vi "Accelerometer Angle.vi"() -> ()   [LabVIEW 2025]
doc: "Accelerometer Example\n\nThis example shows how to use a two axis analog accelerometer to measure angle. The angle of rotation is calculated by taking the inverse tangent of the x-axis value (opposite) over the y-axis value (adjacent). This example does not account for the possible inconsistencies within the accelerometer. The calculation is performed assuming the x-axis and y-axis values form a perfect unit circle.\n\nThis example expects a USB cable connected from your development PC to the Type B USB Jack (next to the power input) on the roboRIO."
uses:
  <vilib>/Rock Robotics/WPI/Accelerometer/WPI_AccelerometerScaling.ctl
  <vilib>/Rock Robotics/WPI/Accelerometer/WPI_AccelerometerAnalogChannels.ctl
  <vilib>/Rock Robotics/SystemInterfaces/AI/FPGA_AIChannel.ctl
  <vilib>/Rock Robotics/WPI/Accelerometer/WPI_AccelerometerAnalogOpen.vi
panel:
  in  "Analog Channels":T1={"X-Axis"=enum."AI 0", "Y-Axis"=enum."AI 1", "Z-Axis"=enum."Invalid"}
  in  "Scaling":T3={"Gain (VoltsPerG)"=1.0, "Center Voltage"=2.5}
  out "Degrees of Rotation":dbl(knob) scale=180.0..-180.0
  in  "stop":bool
  out "Accelerometer Chart":cluster{"Acceleration":dbl, "Acceleration":dbl}(graph)
  # "Set these inputs before running."
  # "If the X axis and Y axis accelerometers are at 90 degrees to each other.  And if they have matching sensitivities.  Then geometry can show that tan(a) = x/y."
  # "This dial illustrates the rotation angle (in degrees) of the x-axis of the accelerometer."
  # "X"
  # "Y"
  # "5"
  # "5"
  # "accelerometer pins"
  # "G"
  # "G"
  # "Y axis"
  # "X axis"
  # "y"
  # "x"
  # "a"
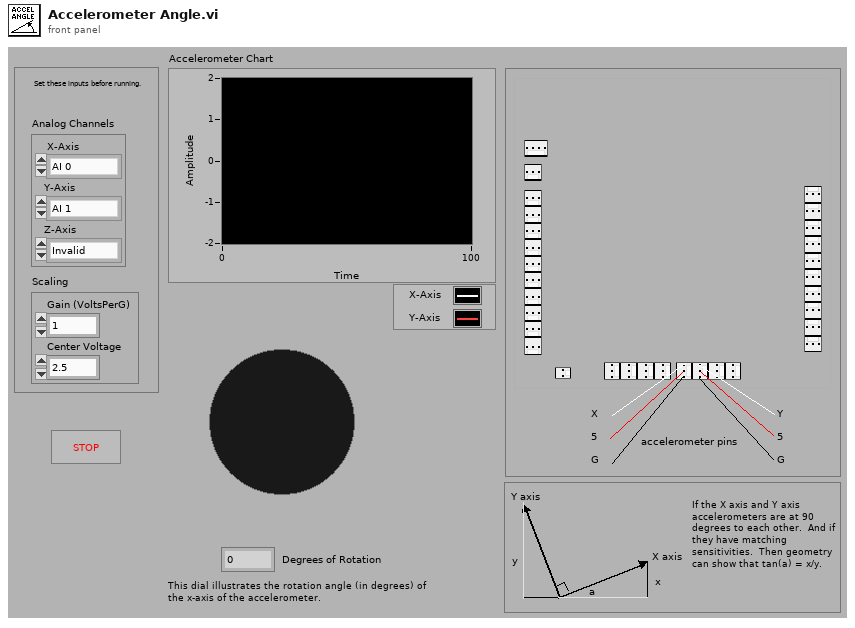
[diagram p1: front panel]
types:
  T1 = typedef "WPI_AccelerometerAnalogChannels.ctl" = cluster{"X-Axis":T2, "Y-Axis":T2, "Z-Axis":T2}
  T2 = typedef "FPGA_AIChannel.ctl" = enum8{"AI 0", "AI 1", "AI 2", "AI 3", "AI MXP 0", "AI MXP 1", "AI MXP 2", "AI MXP 3", "Invalid"}
  T3 = typedef "WPI_AccelerometerScaling.ctl" = cluster{"Gain (VoltsPerG)":dbl, "Center Voltage":dbl}
  T4 = typedef "WPI_AccelerometerDevRef.ctl" = cluster{"DevStatus":errorcluster, "Scaling":T3, "Analog Channels":T1, "I2C Bus":T5, "SPI Bus":T6, "Accel Range":T7, "ADXL Axes":T8, "Handle":i32, "Device Address":u8, "Accel Type":enum16{"Analog", "ADXL345 I2C", "ADXL345 SPI", "Internal", "ADXL362 SPI"}}
  T5 = typedef "i2c_bus.ctl" = enum16{"I2C On-Board", "I2C MXP", "Invalid"}
  T6 = typedef "spi_bus.ctl" = enum16{"SPI On-Board, CS0", "SPI On-Board, CS1", "SPI On-Board, CS2", "SPI On-Board, CS3", "SPI MXP", "Invalid"}
  T7 = typedef "ADXL345 Range.ctl" = u8
  T8 = typedef "WPI_AccelerometerADXL345 Axes.ctl" = cluster{"X-Axis":bool, "Y-Axis":bool, "Z-Axis":bool}
  T9 = cluster{"X-Axis":dbl, "Y-Axis":dbl, "Z-Axis":dbl}
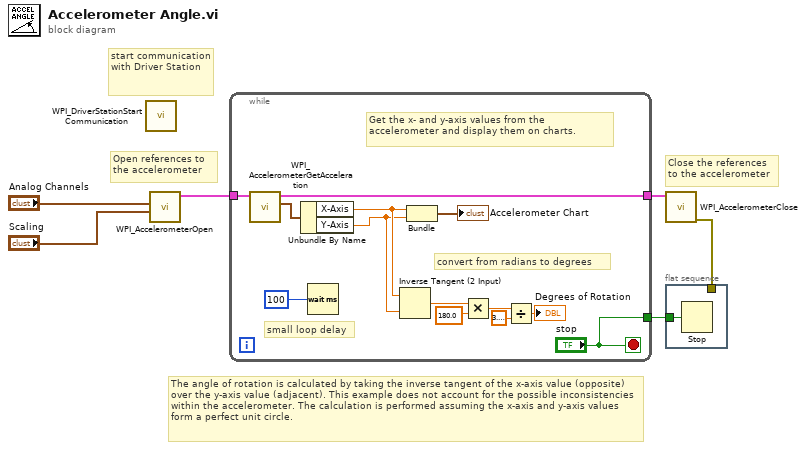
[diagram p0: block diagram]
diagram:
  # "The angle of rotation is calculated by taking the inverse tangent of the x-axis value (opposite) over the y-axis value (adjacent). This example does not account for the possible inconsistencies within the accelerometer. The calculation is performed assuming the x-axis and y-axis values form a perfect unit circle."
  # "start communication with Driver Station"
  # "Close the references\nto the accelerometer"
  # "Open references to \nthe accelerometer"
  n1 = call <vilib>:"WPI_DriverStationStart Communication.vi"() -> ()  [unwired: 3 in, 9 out]
  n2 = call-poly <vilib>:"WPI_AccelerometerOpen.vi"("Scaling"="Scaling", "Analog Channels"="Analog Channels") -> ("AccelerometerDevRef"=w5:T4)  [unwired: 8 in, 1 out]
  n3 = while {
    tunnel: ["stop"] -> w4
    tunnel: [w18] -> w6
    tunnel: w5 -> [w9]
    stop <- "stop" stop-if-true
    # "convert from radians to degrees"
    # "small loop delay"
    # "Get the x- and y-axis values from the accelerometer and display them on charts."
    n4 = call <vilib>:"WPI_AccelerometerGetAcceleration.vi"("AccelerometerDevRef"=w9) -> ("Accelerations"=w11:T9, "AccelerometerDevRef"=w18:T4)  [unwired: 1 in, 8 out]
    n5 = Unbundle By Name(w11) -> ("X-Axis"=w8:dbl, "Y-Axis"=w7:dbl)
    n6 = Wait (ms)(milliseconds to wait=u32 100) -> ()  [unwired: 1 out]
    n7 = Inverse Tangent (2 Input)(1:w7, 2:w8) -> (0:w13:dbl)
    n8 = Bundle("X-Axis"=w8, "Y-Axis"=w7) -> (→"Accelerometer Chart":cluster{"X-Axis":dbl, "Y-Axis":dbl})  [unwired: 1 in]
    n9 = Multiply(x=w13, y=180.0) -> (x*y=w15:dbl)
    n10 = Divide(x=w15, y=3.141592653589793) -> (x/y=→"Degrees of Rotation":dbl)
  }
  n11 = call <vilib>:"WPI_AccelerometerClose.vi"("AccelerometerDevRef"=w6) -> ("error out"=w3:errorcluster)  [unwired: 1 in, 9 out]
  n12 = flat-sequence {
    tunnel: w4 -> [w20]
    tunnel: w3 -> [_]
    frame #0 {
      n13 = Stop(stop? (T)=w20) -> ()
    }
  }
